vi "Script to Tbl.vi"(0 "Script":T1) -> (4 "Tbl":string[][](array[string]))   [LabVIEW 2019]
uses:
  TypeDef/Script.ctl
  TypeDef/Step.ctl
  TypeDef/Direction.ctl
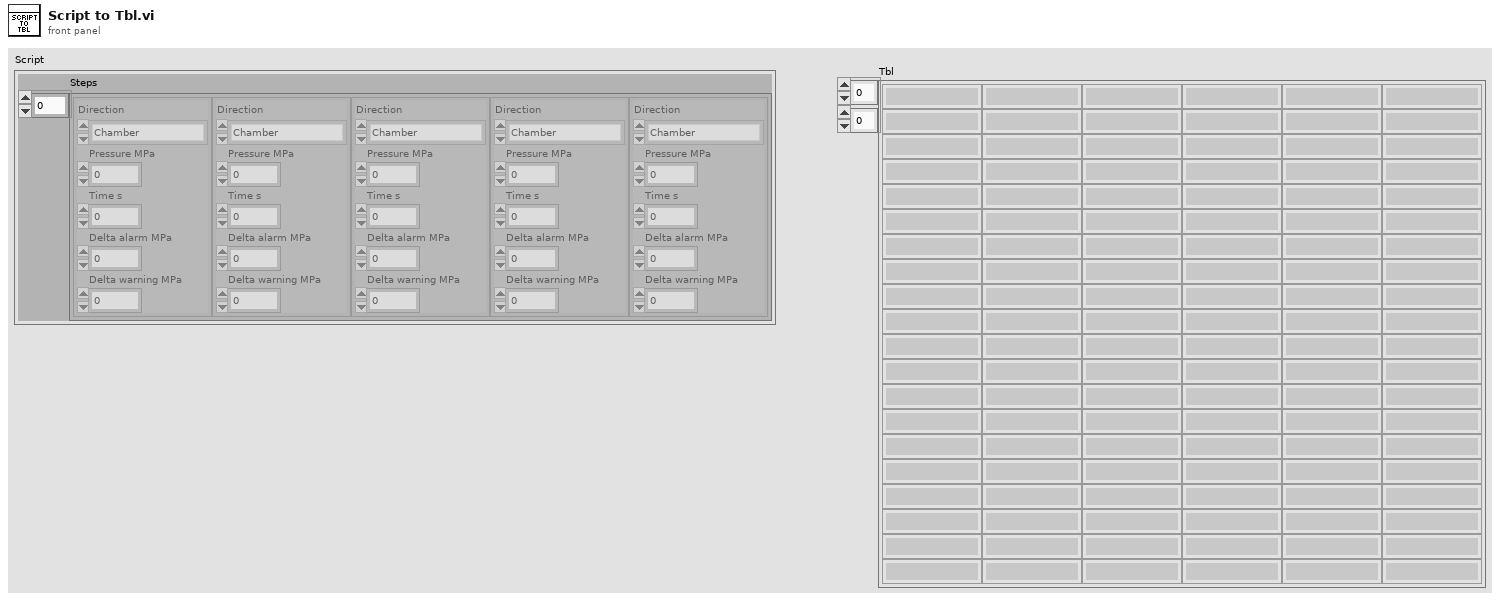
[diagram p1: front panel]
types:
  T1 = typedef "Script.ctl" = cluster{"Steps":T2[]}
  T2 = typedef "Step.ctl" = cluster{"Direction":T3, "Pressure MPa":dbl, "Time s":dbl, "Delta alarm MPa":dbl, "Delta warning MPa":dbl}
  T3 = typedef "Direction.ctl" = enum16{"None", "Chamber", "DUT"}
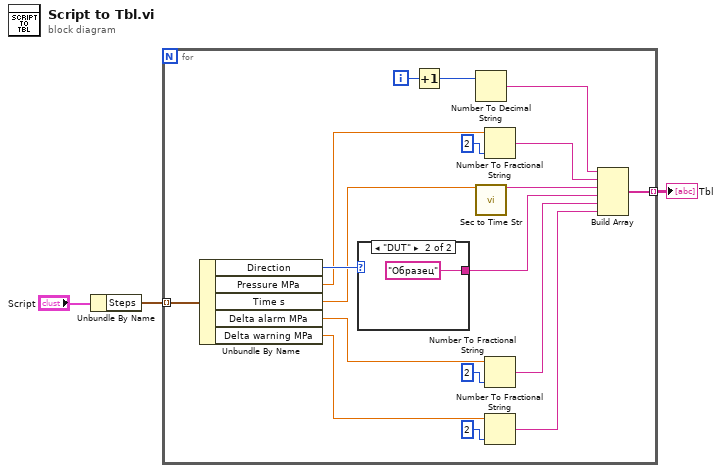
[diagram p0: block diagram]
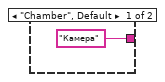
[diagram p2: hidden frame]
diagram:
  n1 = Unbundle By Name("Script") -> ("Steps"=w2:T2[])
  n2 = for {
    tunnel: w2 -> [w21] mode=indexing
    tunnel: [w7] -> w1 mode=indexing
    i -> [w20]
    n3 = Unbundle By Name(w21) -> ("Direction"=w18:T3, "Pressure MPa"=w16:dbl, "Time s"=w14:dbl, "Delta alarm MPa"=w11:dbl, "Delta warning MPa"=w10:dbl)
    n4 = case shown="\"DUT\"" w18 {
      tunnel: ["Камера" "Образец"] -> w4
      frame "Chamber", Default {
      }
      frame "DUT" {
      }
    }
    n5 = Increment(x=w20) -> (x+1=w19:i32)
    n6 = Number To Decimal String(number=w19) -> (decimal integer string=w17:string)  [unwired: 1 in]
    n7 = call "Sec to Time Str.vi"("Time s"=w14) -> ("String"=w5:string)  [unwired: 14 in]
    n8 = Number To Fractional String(number=w16, precision (6)=i16 2) -> (F-format string=w6:string)  [unwired: 2 in]
    n9 = Number To Fractional String(number=w11, precision (6)=i16 2) -> (F-format string=w9:string)  [unwired: 2 in]
    n10 = Number To Fractional String(number=w10, precision (6)=i16 2) -> (F-format string=w8:string)  [unwired: 2 in]
    n11 = Build Array(w17, w6, w5, w4, w9, w8) -> (w7:string[])
  }
  "Tbl" <- w1
